vi "State_Machine.vi"(8 "error in (no error)":errorcluster caption="entrée d'erreur (pas d'erreur)", 11 "Send_Frame en entrée":refnum<class "Nodon_Send_Command_UART.lvclass">) -> (0 "error out":errorcluster caption="sortie d'erreur", 2 "Json_String":string, 3 "Send_Frame en sortie":refnum<class "Nodon_Send_Command_UART.lvclass">)   [LabVIEW 2020, in "Library Test.lvlib" / "Nodon_Send_Command_UART.lvclass"]
uses:
  Nodon_Send_Command_UART.lvclass
  JSON API/Variant JSON/Variant to JSON.vi
  JSON API/JSON Value/Get Item by name array.vi
  JSON API/JSON Value/JSON Value.lvclass
  Nodon_Send_Command_UART.lvclass/Nodon_Send_Command_UART.ctl
  JSON API/Get Polymorphic/JSON GetSet.lvlib
  JSON API/Variant JSON/Variant JSON.lvlib
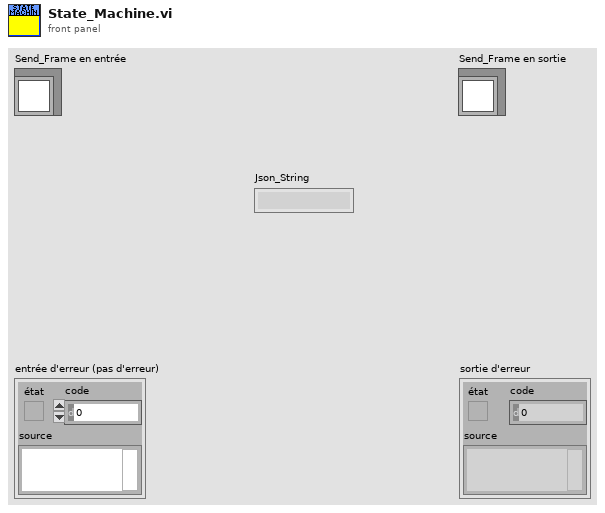
[diagram p1: front panel]
types:
  T1 = cluster{"Commande Type":string, "Command ID":string, "Data":string, "Error":string}
  T2 = enum16{"Empty port", "Send Frame", "Wait Return Ack", "Wait Return Report", "Check End", "End"}
  T3 = enum16{"Empty port", "Send Frame", "Wait Return Ack", "Wait Return Report", "Check End"}
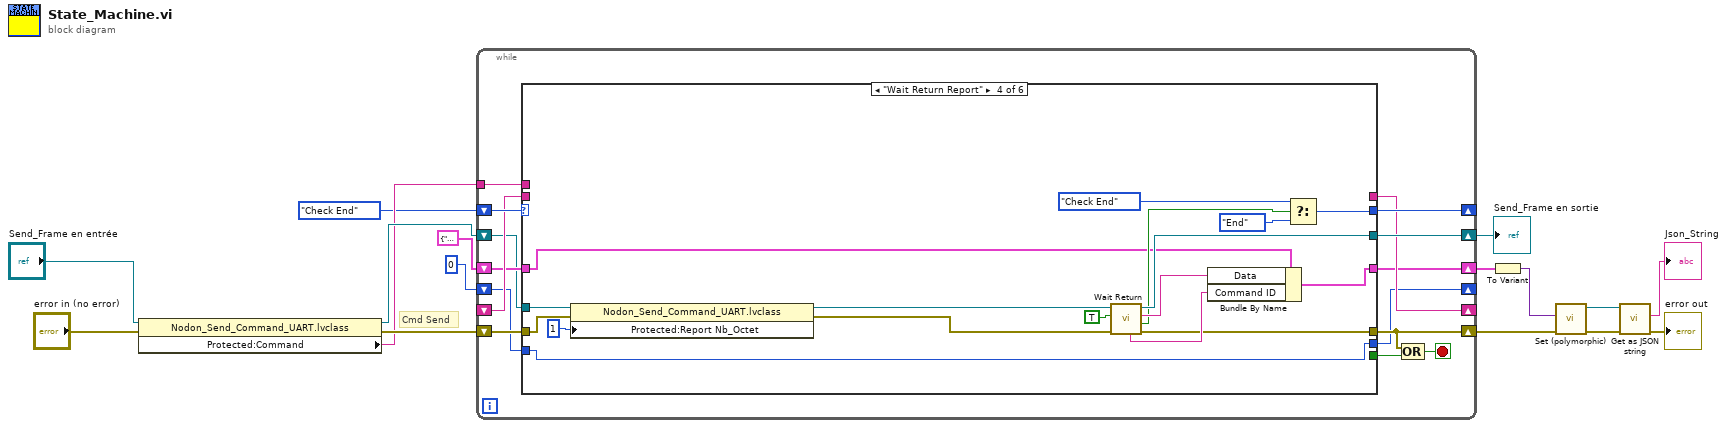
[diagram p0: block diagram]
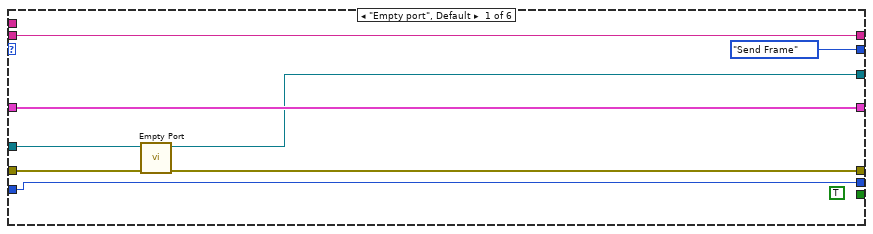
[diagram p2: hidden frame]
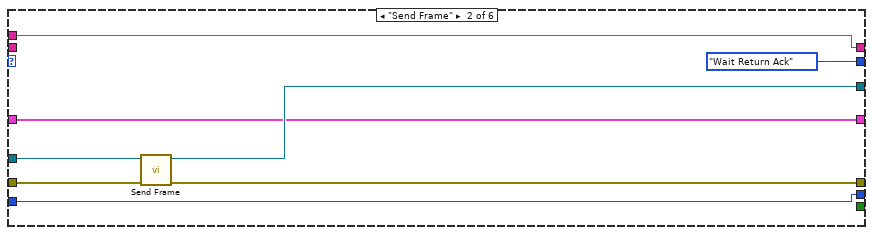
[diagram p3: hidden frame]
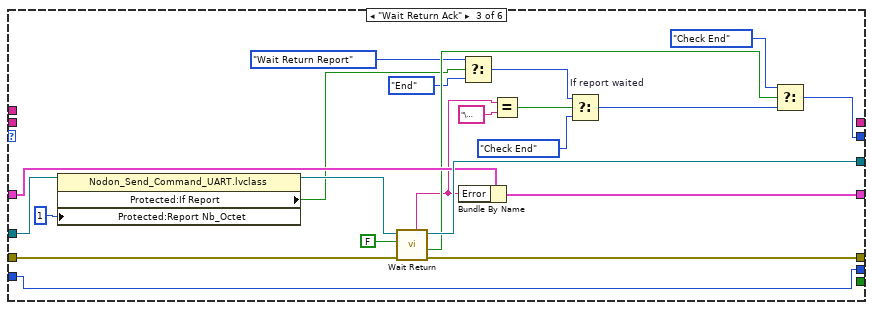
[diagram p4: hidden frame]
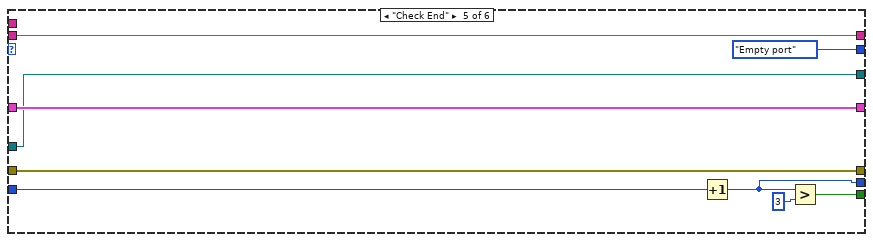
[diagram p5: hidden frame]
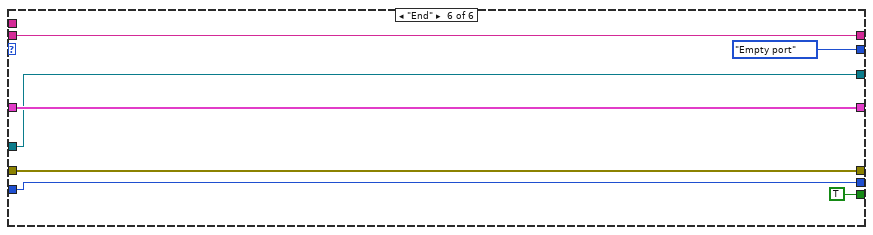
[diagram p6: hidden frame]
diagram:
  # "Cmd Send"
  n1 = property class="Nodon_Send_Command_UART.lvclass"(reference="Send_Frame en entrée", error in="error in (no error)") -> (reference out=w14:refnum<class "Nodon_Send_Command_UART.lvclass">, error out=w13:errorcluster, "Protected:Command"=w11:string)
  n2 = while {
    tunnel: w11 -> [w30]
    shift-right: [w31] -> w15
    shift-left: w14 -> [w22]
    shift-right: [w21] -> w3
    shift-left: w13 -> [w29]
    shift-right: [w28] -> _
    shift-left: T2."Check End" -> [w27]
    shift-right: [w25] -> _
    shift-left: _ -> [w26]
    shift-right: [w23] -> w2
    shift-left: T1 {"Commande Type"="", "Command ID"="", "Data"="", "Error"=""} -> [w24]
    shift-right: [w17] -> _
    shift-left: 0 -> [w19]
    stop <- w20 stop-if-true
    n3 = case shown="\"Wait Return Report\"" w27 {
      tunnel: [w37 w47 w63 w80 w95 w102] -> w21
      tunnel: [w34 w46 w68 w86 w91 w98] -> w31
      tunnel: w30 -> [_ w44 _ _ _ _]
      tunnel: w29 -> [w39 w45 w69 w79 w95 w102]
      tunnel: [T2."Send Frame" T2."Wait Return Ack" w67 w85 T3."Empty port" T3."Empty port"] -> w28
      tunnel: [w38 w44 _ _ w94 w101] -> w25
      tunnel: w26 -> [w38 _ _ _ w94 w101]
      tunnel: w24 -> [w36 w43 w64 w70 w92 w99]
      tunnel: [w36 w43 w65 w81 w92 w99] -> w23
      tunnel: w22 -> [w35 w42 w62 w78 w91 w98]
      tunnel: w19 -> [w32 w40 w49 w72 w88 w96]
      tunnel: [_ _ _ _ w89 TRUE] -> w18
      tunnel: [w32 w40 w49 w72 w87 w96] -> w17
      frame "Empty port", Default {
        (unwired) TRUE ("Frame NOk")
        n4 = call-dynamic "Empty Port.vi"("entrée d'erreur (pas d'erreur)"=w39, "Send_Frame en entrée"=w35) -> ("sortie d'erreur"=w37:errorcluster, "Send_Frame en sortie"=w34:refnum<class "Nodon_Send_Command_UART.lvclass">)  [unwired: 8 in]
      }
      frame "Send Frame" {
        n5 = call-dynamic "Send Frame.vi"("entrée d'erreur (pas d'erreur)"=w45, "Send_Frame en entrée"=w42) -> ("sortie d'erreur"=w47:errorcluster, "Send_Frame en sortie"=w46:refnum<class "Nodon_Send_Command_UART.lvclass">)  [unwired: 8 in]
      }
      frame "Wait Return Ack" {
        n6 = property class="Nodon_Send_Command_UART.lvclass"(reference=w62, "Protected:Report Nb_Octet"=u16 1 ("Report Nb_Octet")) -> (reference out=w61:refnum<class "Nodon_Send_Command_UART.lvclass">, "Protected:If Report"=w53:bool)  [unwired: 1 in, 1 out]
        n7 = call-dynamic "Wait Return.vi"("entrée d'erreur (pas d'erreur)"=w69, "Report ?"=FALSE ("Report"), "Send_Frame en entrée"=w61) -> ("sortie d'erreur"=w63:errorcluster, "Send again"=w56:bool, "Send_Frame en sortie"=w68:refnum<class "Nodon_Send_Command_UART.lvclass">, "Command Type"=w48:string)  [unwired: 3 in, 2 out]
        n8 = Bundle By Name(cluster=w64, "Error"=w48) -> (w65:T1)
        n9 = Select(t=T2."Wait Return Report", s=w53, f=T2."End") -> (s? t:f=w51:T2)
        n10 = Equal?(x=w48, y="\u0000") -> (x = y?=w58:bool)
        n11 = Select "If report waited"(t=w51, s=w58, f=T2."Check End") -> (s? t:f=w57:T2)
        n12 = Select(t=T2."Check End", s=w56, f=w57) -> (s? t:f=w67:T2)
      }
      frame "Wait Return Report" {
        n13 = property class="Nodon_Send_Command_UART.lvclass"(reference=w78, error in=w79, "Protected:Report Nb_Octet"=u16 1 ("Report Nb_Octet")) -> (reference out=w77:refnum<class "Nodon_Send_Command_UART.lvclass">, error out=w71:errorcluster)
        n14 = call-dynamic "Wait Return.vi"("entrée d'erreur (pas d'erreur)"=w71, "Report ?"=TRUE ("Report"), "Send_Frame en entrée"=w77) -> ("sortie d'erreur"=w80:errorcluster, "Send again"=w75:bool, "Data"=w82:string, "Send_Frame en sortie"=w86:refnum<class "Nodon_Send_Command_UART.lvclass">, "Command ID"=w83:string)  [unwired: 3 in, 1 out]
        n15 = Bundle By Name(cluster=w70, "Data"=w82, "Command ID"=w83) -> (w81:T1)
        n16 = Select(t=T2."Check End", s=w75, f=T2."End") -> (s? t:f=w85:T2)
      }
      frame "Check End" {
        n17 = Increment(x=w88) -> (x+1=w87:i32)
        n18 = Greater?(x=w87, y=3) -> (0:w89:bool)
      }
      frame "End" {
      }
    }
    n19 = Compound Arithmetic op=OR ("Opérateur arithmétique")(w21, w18) -> (w20:bool)
  }
  "Send_Frame en sortie" <- w15
  n20 = To Variant(anything=w2) -> (Variant=w4:variant)
  n21 = call-poly "Set (polymorphic).vi"("error in (no error)"=w3, "Variant"=w4) -> ("error out"=w6:errorcluster, "JSON Value out"=w5:refnum<class "JSON Value.lvclass">)  [unwired: 8 in]
  n22 = call "Get as JSON string.vi"("error in (no error)"=w6, "JSON Value in"=w5) -> ("error out"=→"error out":errorcluster, "<JSON>"=→"Json_String":string)  [unwired: 8 in]
